vi "Subscribe (async).vi"(8 "error in (no error)":errorcluster, 9 "Topic":string, 11 "WAMP Client in":refnum<class "WAMP Client.lvclass">) -> (0 "error out":errorcluster, 2 "notifier out":refnum<notifier>, 3 "WAMP Client out":refnum<class "WAMP Client.lvclass">)   [LabVIEW 2020, in "wamplv.lvlib" / "WAMP Client.lvclass"]
uses:
  WAMP Client.lvclass
  TypeDef/Subscribe Result.ctl
  TypeDef/EVENT payload.ctl
  API/TypeDefs/Combined error.ctl
  API/TypeDefs/WAMP error.ctl
  TypeDef/SUBSCRIBE Request Data.ctl
  TypeDef/Internal Message Type.ctl
  WAMP Client.lvclass/WAMP Client.ctl
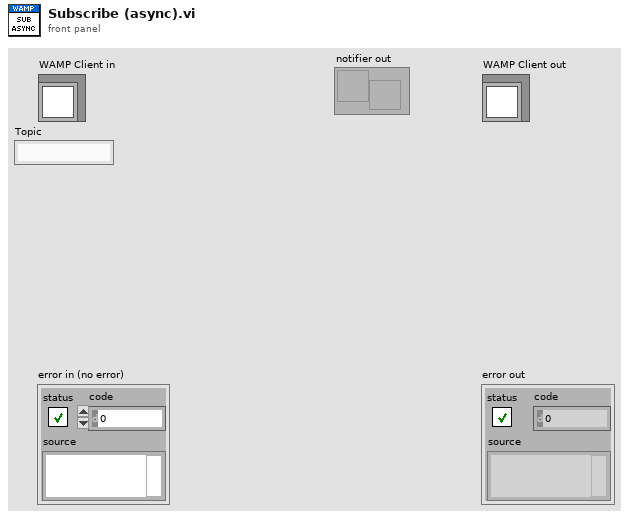
[diagram p1: front panel]
types:
  T1 = typedef "wamplv.lvlib/WAMP Client.lvclass/Subscribe Result.ctl" = cluster{"Success?":bool, "Publication Received Event":refnum<user-event>, "Combined Error":T2}
  T2 = typedef "wamplv.lvlib/WAMP Client.lvclass/Combined error.ctl" = cluster{"Error?":bool, "WAMP Error":T3, "Error":errorcluster}
  T3 = typedef "wamplv.lvlib/WAMP Client.lvclass/WAMP error.ctl" = cluster{"Details":string, "ArgumentKw Payload":string, "Error?":bool, "Error URI":string, "Arguments Payload":string}
  T4 = typedef "wamplv.lvlib/WAMP Client.lvclass/Internal Message Type.ctl" = enum16{"Subscribe", "Handle Subscribed", "Handle Event", "Unsubscribe", "Handle Unsubscribed", "Publish", "Handled Published", "Goodbye", "Handle Goodbye", "Call", "Handle Result", "Register", "Handle Registered", "Unregister", "Handle Unregistered", "Handle Invocation", "Yield", "Error"}
  T5 = typedef "wamplv.lvlib/WAMP Client.lvclass/SUBSCRIBE Request Data.ctl" = cluster{"Topic":string, "Subscribe result notifer":refnum<notifier>}
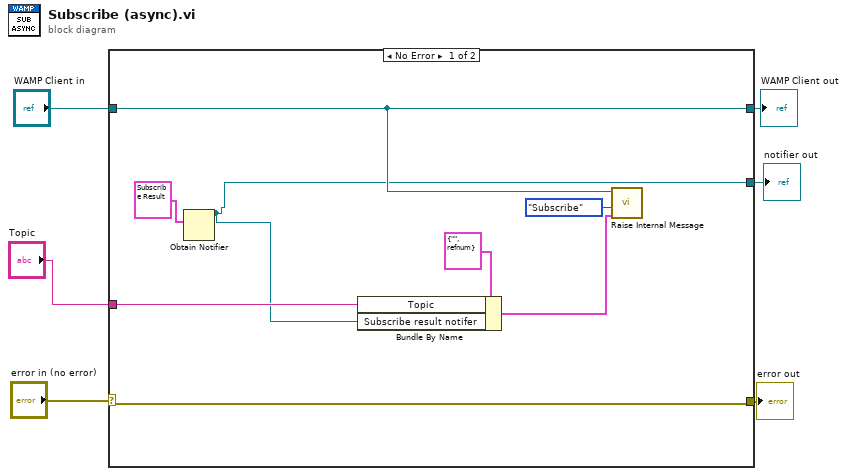
[diagram p0: block diagram]
diagram:
  n1 = case shown="No Error" "error in (no error)" {
    selector: "error in (no error)" -> [w14 w16]
    tunnel: [w14 w16] -> w5
    tunnel: [w13 w15] -> w3
    tunnel: "WAMP Client in" -> [w13 w15]
    tunnel: "Topic" -> [w10 _]
    tunnel: [w8 _] -> w1
    frame No Error {
      n2 = Obtain Notifier(notification data type=T1 {"Success?"=FALSE, "Publication Received Event"=refnum, "Combined Error"={"Error?"=FALSE, "WAMP Error"={"Details"="", "ArgumentKw Payload"="{}", "Error?"=FALSE, "Error URI"="", "Arguments Payload"=""}, "Error"={"status"=FALSE, "code"=0, "source"=""}}} ("Subcsribe Result")) -> (notifier out=w8:refnum<notifier>)  [unwired: 3 in, 2 out]
      n3 = Bundle By Name(cluster=T5 {"Topic"="", "Subscribe result notifer"=refnum} ("Cluster"), "Topic"=w10, "Subscribe result notifer"=w8) -> (w11:T5)
      n4 = call-dynamic "Raise Internal Message.vi"("Variant"=w11, "Internal Message Type"=Internal_Message_Type."Subscribe", "WAMP Client in"=w13) -> ()  [unwired: 7 in, 2 out]
    }
    frame Error {
    }
  }
  "error out" <- w5
  "WAMP Client out" <- w3
  "notifier out" <- w1
